vi "质控中断报警全局.vi"() -> ()   [LabVIEW 2016, in "质控单元.lvlib"]
panel:
  out "总氮传感器故障报警":bool
  out "CODCr传感器故障报警":bool
  out "CODMn传感器故障报警":bool
  out "总磷传感器故障报警":bool
  out "氨氮传感器故障报警":bool
  in  "CODCr中断报警":bool
  in  "CODMn中断报警":bool
  in  "总氮中断报警":bool
  in  "总磷中断报警":bool
  in  "氨氮中断报警":bool
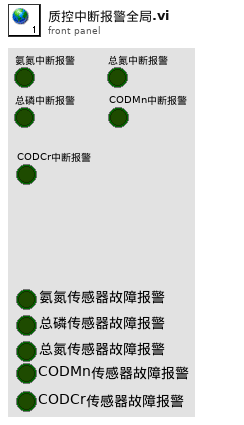
[diagram p1: front panel]
diagram:
